vi "Lockin-4461_Multiple Inputs and Outputs_KH_functional_global_waveform.vi"(8 "stop":bool) -> ()   [LabVIEW 2013]
uses:
  <vilib>/Analysis/4window.llb/windowTd.ctl
  <vilib>/Analysis/3filter.llb/Filter Structure Type.ctl
  <vilib>/Analysis/baseanly.llb/Mean (DBL).vi
  <vilib>/Analysis/2dsp.llb/Decimate (single shot, DBL).vi
  <vilib>/DAQmx/write.llb/DAQmx Write (Analog 1D Wfm NChan NSamp).vi
  DAQ-Lockin-SubVI/Lock-in Globles Multiple Inputs and Outputs used with FGV.vi
  <vilib>/DAQmx/miscellaneous.llb/DAQmx Fill In Error Info.vi
  <vilib>/measure/macond.llb/IIR Filter for N Chan.vi
  <vilib>/measure/madcrms.llb/Basic Averaged DC-RMS for N Chan.vi
  <vilib>/measure/maspectr.llb/FFT Power Spectrum and PSD for N Chan.vi
  <vilib>/Analysis/NI_AALPro.lvlib
  <vilib>/Analysis/NI_AALBase.lvlib
  <vilib>/measure/NI_MAPro.lvlib
  <vilib>/measure/NI_MABase.lvlib
panel:
  out "phase log":dbl[](array[numeric])=[0.9999999998974775, 0.9999999998974775, 0.9999999998974775, 0.9999999998974775]
  in  "Input Signals":i16(slide)=2 scale=1.0..20.0
  in  "Tab Control 2":T1(tab)=enum."Lock-in Settings"
  in  "Auto control  max AI rate/ AI block size":bool=TRUE
  in  "AI Buffer Size (S)":i32=10
  in  "AI Block Size":i32=14350
  out "AI Rate":dbl=193151.0 format="%.2f"
  in  "AI Configuration":T2(array[cluster])=[{"AI.Coupling"=10050, "AI.Max"=10.0, "AI.Min"=-10.0, "Input physical channels"="PXI1Slot2/ai0:1"}, {"AI.Coupling"=10050, "AI.Max"=10.0, "AI.Min"=-10.0, "Input physical channels"="PXI1Slot3/ai0:1"}, {"AI.Coupling"=10050, "AI.Max"=10.0, "AI.Min"=-10.0, "Input physical channels"="PXI1Slot5/ai0:1"}, {"AI.Coupling"=10050, "AI.Max"=10.0, "AI.Min"=-10.0, "Input physical channels"="PXI1Slot6/ai0:1"}] {"AI.Coupling" items=["AC"=10045, "DC"=10050, "GND"=10066]}
  in  "AO Configuration":T3(array[cluster])=[{"Output physical channels"="PXI1Slot2/ao0:1", "AO. Max"=0.1, "AO.Min"=-0.1}, {"Output physical channels"="PXI1Slot3/ao0:1", "AO. Max"=0.25, "AO.Min"=-0.25}, {"Output physical channels"="PXI1Slot5/ao0:1", "AO. Max"=0.1, "AO.Min"=-0.1}, {"Output physical channels"="PXI1Slot6/ao0:1", "AO. Max"=0.1, "AO.Min"=-0.1}]
  in  "OSC Configuration":T4(array[cluster])=[[{"Signal Type"=enum."Sine Wave", "DC"=0.0, "Amplitude"=0.0, "frequency"=13.46, "Phase"=0.0}, {"Signal Type"=enum."Sine Wave", "DC"=0.0, "Amplitude"=0.0005, "frequency"=13.46, "Phase"=0.0}], [{"Signal Type"=enum."Sine Wave", "DC"=0.0, "Amplitude"=0.0, "frequency"=13.46, "Phase"=0.0}, {"Signal Type"=enum."Sine Wave", "DC"=0.0, "Amplitude"=0.0, "frequency"=13.46, "Phase"=0.0}], [{"Signal Type"=enum."Sine Wave", "DC"=0.0, "Amplitude"=0.0, "frequency"=13.46, "Phase"=0.0}, {"Signal Type"=enum."Sine Wave", "DC"=0.0, "Amplitude"=0.0, "frequency"=13.46, "Phase"=0.0}], [{"Signal Type"=enum."Sine Wave", "DC"=-0.0467, "Amplitude"=0.0, "frequency"=13.46, "Phase"=0.0}, {"Signal Type"=enum."Sine Wave", "DC"=0.0, "Amplitude"=0.0, "frequency"=13.46, "Phase"=0.0}]] {"frequency" step=0.001 format="%.3p"; "Amplitude" format="%0.2p"; "DC" min=-0.99 max=0.99 format="%.2p"}
  in  "Phase&Tc":T5(array[cluster])=[{"Phase"=0.0, "Time constant"=0.5, "Set Tc"=FALSE, "Autophase"=FALSE, "Order"=0.0}, {"Phase"=0.0, "Time constant"=0.5, "Set Tc"=FALSE, "Autophase"=FALSE, "Order"=0.0}, {"Phase"=0.0, "Time constant"=0.5, "Set Tc"=FALSE, "Autophase"=FALSE, "Order"=0.0}, {"Phase"=0.0, "Time constant"=0.5, "Set Tc"=FALSE, "Autophase"=FALSE, "Order"=0.0}, {"Phase"=0.0, "Time constant"=0.5, "Set Tc"=FALSE, "Autophase"=FALSE, "Order"=0.0}, {"Phase"=0.0, "Time constant"=0.5, "Set Tc"=FALSE, "Autophase"=FALSE, "Order"=0.0}, {"Phase"=0.0, "Time constant"=0.5, "Set Tc"=FALSE, "Autophase"=FALSE, "Order"=0.0}, {"Phase"=0.0, "Time constant"=0.5, "Set Tc"=FALSE, "Autophase"=FALSE, "Order"=0.0}] {"Phase" min=0.0 max=360.0 scale=0.0..360.0}
  in  "Gain":dbl[](array[numeric])=[0.001, 2e-08, 0.001, 0.001, 0.001, 2e-08]
  in  "frequency":dbl
  out "max ai rate":i32=200000
  in  "zero offset":bool
  in  "measure offset":bool
  out "elapsed time":dbl format="%.2g"
  out "Display 2":string="-189.706780      pA"
  out "Display 1":string="-  1.195069      nA"
  in  "Remote":bool=TRUE
  in  "Display":u16(ring) items=["X and Y", "R and Theta"]
  out "Backlog":u8(slide) scale=0.0..100.0
  out "Sampling information":cluster{"Fs":dbl, "#s":dbl}[](array[cluster])=[{"Fs"=193151.0, "#s"=14350.0}, {"Fs"=193151.0, "#s"=14350.0}, {"Fs"=193151.0, "#s"=14350.0}, {"Fs"=193151.0, "#s"=14350.0}]
  out "AO Task":refnum<k21>[](array[refnum])
  out "AI task":refnum<k21>[](array[refnum])
  in  "Tab Control":T6(tab)=enum."Input signals"
  out "Display X (or R) A":dbl[](graph)=[0.0003515597766155211, 0.0003507181675748926, 0.00035141371795365553, 0.0003511676429896116, 0.00035187230028368424, 0.00035142951363845783, 0.00035200218342147584, 0.0003516475669745772, 0.0003513264804061819, 0.0003512466291338144, 0.00035057064868592705, 0.0003509796679868739, 0.0003503537452691344, 0.00035135722504198624, 0.0003499281739531895, 0.00035086727974118317, 0.00035123877543565506, 0.00035105622304100427, 0.00035125795255371527, 0.00035135096570343606, 0.00035150903711195496, 0.0003505963637110228, 0.00035169258826266966, 0.00035039322315619063, 0.00035053162210950205, 0.00034979480515196903, 0.00035116833497217555, 0.00035144449100699994, 0.0003510879884516026, 0.00035159349196440626, 0.0003508268451218459, 0.0003511494372195583, 0.0003501864505254134, 0.00035068434585759, 0.0003499157469483272, 0.00035133561940496534, 0.0003501980965627419, 0.0003508062229105727, 0.0003512488754734741, 0.00035101108207568276, 0.000350758527959875, 0.0003505205072637121, 0.0003508151287793871, 0.0003508447380896511, 0.0003507555783012489, 0.0003502437335620398, 0.00035109131124810123, 0.0003498450741887054, 0.00035085670677781735, 0.00034947118732054223, 0.0003511126940251815, 0.0003498712344731183, 0.00035107848043918404, 0.00035092762190149656, 0.00035131019104293144, 0.00035117278992843757, 0.00035060771724494964, 0.00035097354822363525, 0.00034979186802935094, 0.0003511746212457802, 0.0003504305912612818, 0.0003514156401972867, 0.0003503117115571819, 0.0003512893859642446, 0.0003509935260745274, 0.0003513343838004985, 0.00035176841277986657, 0.0003515970316337863, 0.0003513166742771524, 0.00035104054487817416, 0.0003513553972404074, 0.0003509590909684851, 0.00035237906837522605, 0.00034999762062152867, 0.00035101065218240423, 0.0003504366384126203, 0.00035118217997485036, 0.00035142807787819834, 0.00035048373763264237, 0.00035091253545080304, 0.00035015216674575555, 0.00035129179836784774, 0.00035001054715737636, 0.0003513927563841236, 0.0003506721750452684, 0.00035171243027286867, 0.0003514132808403294, 0.00035144774997313054, 0.00035154044709008854, 0.0003519234717441954, 0.0003516730726749858, 0.0003510679416845872, 0.00035125236026625956, 0.0003506717477152614, 0.00035179090850881385, 0.00035059443995565375, 0.0003512356648576366, 0.00035099014639157884, 0.00035160877389527615, 0.0003511922254044786, 0.0003522473208559999, 0.000351701222721286, 0.00035138480038931065, 0.0003513741316379797, 0.0003514851249003675, 0.00035153133788109374, 0.00035099743725480883, 0.0003517112066303713, 0.00035087507155982204, 0.0003514136294778693, 0.00035113141545342375, 0.0003516959886248813, 0.00035089134479069386, 0.00035195932575444284, 0.0003510852464980746, 0.00035095112846043197, 0.00035142787266349444, 0.00035033572449709563, 0.0003518389763278957, 0.0003509974314077956, 0.0003521376695816606, 0.0003512642342070748, 0.00035127618489995405, 0.0003514483445065015, 0.00035163795610624693, 0.00035111410128884024, 0.0003509321167631999, 0.0003510796360339337, 0.0003503292989579528, 0.00035156402647202597, 0.0003512873517971787, 0.00035157967118798955, 0.0003510116552725674, 0.00035141232666041183, 0.00035107492263834197, 0.0003512565883348785, 0.0003508476519342546, 0.00035108010765180813, 0.0003516328893962722, 0.00035126967501414075, 0.00035163302601165687, 0.0003503689014483799, 0.00035132816396016856, 0.00035068072793987285, 0.00035165998148334955, 0.0003506716705224395, 0.00035129129082704685, 0.0003506971941344991, 0.000350963932032198, 0.00035118513223693614, 0.00035074827788279046, 0.0003510020040280428, 0.0003504848068533489, 0.0003513321853419367, 0.0003503106012231704, 0.00035095822008976673, 0.0003502387857211528, 0.00035109477850426885, 0.0003507864147016284, 0.00035140137858089053, 0.0003514994969105284, 0.0003513918557124627, 0.0003513696821528527, 0.0003508483346289989, 0.0003515212484504822, 0.0003510208186503463, 0.00035172200150656446, 0.00035110641441137973, 0.00035150387093385414, 0.000351046214234429, 0.0003512959219150425, 0.00035191226359241245, 0.0003519236956018965, 0.0003521320087141144, 0.00035099481829272187, 0.00035189540980659097, 0.00035122584644459046, 0.00035158482485956113, 0.0003502803891156385, 0.00035140356164375307, 0.0003509192077086382, 0.0003516851651443288, 0.00035113340325199413, 0.0003512155559510749, 0.0003512258338077835, 0.0003520237023195563, 0.00035088778042110256, 0.00035164083859914543, 0.0003511937863128998, 0.0003518097746241161, 0.0003512714055365024, 0.000352054622085523, 0.0003513780489555605, 0.0003520135769537603, 0.00035157613181737254, 0.0003514540449784146, 0.00035148596975263194, 0.00035058490211263083, 0.0003514386933989605, 0.0003509759320918032]
  out "Display Y (or Theta) A":dbl[](graph)=[-6.733399539668474e-05, -6.542411496845478e-05, -6.796694874685229e-05, -6.507135674382902e-05, -6.76731893269279e-05, -6.432724937539189e-05, -6.686858480018215e-05, -6.439302698787755e-05, -6.743074524483553e-05, -6.5540559290562e-05, -6.769912727311773e-05, -6.675855899422707e-05, -6.556455830757394e-05, -6.791926016049456e-05, -6.499870275650685e-05, -6.76094096444829e-05, -6.409372415827203e-05, -6.690358743848511e-05, -6.376319395976735e-05, -6.661678688045064e-05, -6.475221640770524e-05, -6.767037729114109e-05, -6.65568517718371e-05, -6.61078983653106e-05, -6.72090065494324e-05, -6.491767883192775e-05, -6.840639245595013e-05, -6.446292181235111e-05, -6.733865135996714e-05, -6.40653784901512e-05, -6.70766205814384e-05, -6.448431014524983e-05, -6.721244620921082e-05, -6.59878655486392e-05, -6.692322551150028e-05, -6.69019264583306e-05, -6.53521862403277e-05, -6.794558923933263e-05, -6.499376607325872e-05, -6.696965991750598e-05, -6.461599929467364e-05, -6.687775724991745e-05, -6.35960014145792e-05, -6.71748832581576e-05, -6.492398900048032e-05, -6.746798157246069e-05, -6.634689247733003e-05, -6.592248825579343e-05, -6.76983125588508e-05, -6.466202421410609e-05, -6.750345332833928e-05, -6.450271804110632e-05, -6.73820213196671e-05, -6.398878990855814e-05, -6.699882608984017e-05, -6.499280498169577e-05, -6.738425010553764e-05, -6.660128249440328e-05, -6.641623559943719e-05, -6.741839015150833e-05, -6.490399197802229e-05, -6.807262637843706e-05, -6.461095964170923e-05, -6.741693933791136e-05, -6.396241139824065e-05, -6.68953533836962e-05, -6.437486412654718e-05, -6.719672530343625e-05, -6.601025951582242e-05, -6.755243507643756e-05, -6.683904754234452e-05, -6.581328668735525e-05, -6.7956730495926e-05, -6.454210702322087e-05, -6.700846714162137e-05, -6.487036358948187e-05, -6.717145047610366e-05, -6.394657730710213e-05, -6.721398561579939e-05, -6.542844878392274e-05, -6.72242800275423e-05, -6.601836591155777e-05, -6.679640312152599e-05, -6.724964008795247e-05, -6.524389201445212e-05, -6.81709788892876e-05, -6.504870506524659e-05, -6.716417310946288e-05, -6.469364606167295e-05, -6.64118927639841e-05, -6.428422401809015e-05, -6.726075100677492e-05, -6.602001398773281e-05, -6.684946783051746e-05, -6.665356018961591e-05, -6.559302821306713e-05, -6.823961541895857e-05, -6.489902378019219e-05, -6.747231633806965e-05, -6.460461787722171e-05, -6.739619325891061e-05, -6.42568749063365e-05, -6.728357578332122e-05, -6.572581320455293e-05, -6.733133575279844e-05, -6.745384605205556e-05, -6.654768580556922e-05, -6.752884945881219e-05, -6.516474446690376e-05, -6.800609459823608e-05, -6.47878614014136e-05, -6.730160658797204e-05, -6.420250070636625e-05, -6.676581343835398e-05, -6.447454426249553e-05, -6.739644425949934e-05, -6.633928104016707e-05, -6.668506011610336e-05, -6.704708770176857e-05, -6.518924517552728e-05, -6.80110716513718e-05, -6.449044290923919e-05, -6.713463098761624e-05, -6.431427908560736e-05, -6.666702370071547e-05, -6.380160055564429e-05, -6.69295226583365e-05, -6.559831844106169e-05, -6.733302905782082e-05, -6.676258268638944e-05, -6.581664753168712e-05, -6.791627178025961e-05, -6.483985086130437e-05, -6.771582429628417e-05, -6.456692771022534e-05, -6.710554331363558e-05, -6.416205680544463e-05, -6.721382973122853e-05, -6.497521331755278e-05, -6.762221774081424e-05, -6.644148745970977e-05, -6.650204706057299e-05, -6.779409446006897e-05, -6.513429971844772e-05, -6.716283035881229e-05, -6.500520220536936e-05, -6.748818593189037e-05, -6.375021526081944e-05, -6.679304519274533e-05, -6.44009832356367e-05, -6.697029619860621e-05, -6.614507717764695e-05, -6.675045380090485e-05, -6.699368958403159e-05, -6.540977419016514e-05, -6.751824094235534e-05, -6.497224203386006e-05, -6.747996187391402e-05, -6.445371747351958e-05, -6.694216412544935e-05, -6.39145549472495e-05, -6.67208337122775e-05, -6.499887641961741e-05, -6.75636406906266e-05, -6.646187561893783e-05, -6.6422353672184e-05, -6.774188283466967e-05, -6.49718493653088e-05, -6.774060340062207e-05, -6.447729538855726e-05, -6.7276329542447e-05, -6.45413468122233e-05, -6.725796598454556e-05, -6.43215545435326e-05, -6.710426281533913e-05, -6.640793922515245e-05, -6.688725807556598e-05, -6.702595030422637e-05, -6.555532275656158e-05, -6.775334049196785e-05, -6.485489689304207e-05, -6.778283710493148e-05, -6.47406497658257e-05, -6.667061103568536e-05, -6.71178176816977e-05, -6.545036016336727e-05, -6.758648874374465e-05, -6.648186107488955e-05, -6.564351224820166e-05, -6.726344507999936e-05, -6.562770441403993e-05, -6.793015780847218e-05, -6.469220243177453e-05, -6.740767551952607e-05, -6.44720529171589e-05, -6.682838905210087e-05, -6.483406975990464e-05, -6.710332224721377e-05, -6.629467593853179e-05, -6.657765389063085e-05]
  in  "long term averaging type":enum16{"Linear", "Exponential"}(ring)
  in  "averaging type":enum16{"Linear", "Exponential"}(ring)
  out "Waveform Graph":waveform(dbl)[](graph)
  in  "Stream to disk?":bool
  in  "decimating factor":i32
  in  "decimating factor 2":i32=1
  out "Waveform Graph 2":cluster{"f0":dbl, "df":dbl, "magnitude":dbl[]}[](graph)
  in  "window":T7=1 items=["Rectangle"=0, "Hanning"=1, "Hamming"=2, "Blackman-Harris"=3, "Exact Blackman"=4, "Blackman"=5, "Flat Top"=6, "4 Term B-Harris "=7, "7 Term B-Harris"=8, "Low Sidelobe"=9, "Blackman Nuttall"=11, "Triangle"=30, "Bartlett-Hanning"=31, "Bohman"=32, "Parzen"=33, "Welch"=34, "Kaiser"=60, "Dolph-Chebyshev"=61, "Gaussian"=62]
  in  "averaging parameters":T8={"averaging mode"=enum."No averaging", "weighting mode"=enum."Exponential", "number of averages"=10} {"number of averages" min=1}
  in  "dB On (F)":bool
  out "Results (X, Y, R, Theta)":dbl[][](array[numeric]) format="%#_6p"
  out "Measure?":u16[](array[numeric])=[2, 1, 2, 2, 2, 1]
  in  "Cluster (unused right now)":T9={"Amplitude"=[0.001, 2e-08, 0.001, 0.001, 0.001, 2e-08], "DC"=[0.001, 2e-08, 0.001, 0.001, 0.001, 2e-08], "phase"=[0.001, 2e-08, 0.001, 0.001, 0.001, 2e-08], "Array"=[]}
  out "offsets":dbl[](array[numeric])
  in  "IIR filter specifications":T10={"Topology"=enum."Butterworth", "Type"=enum."Lowpass", "Order"=1, "Lower Fc"=100.0, "Upper Fc"=200.0, "PB Ripple"=1.0, "SB Attenuation"=60.0} {"PB Ripple" format="%0.2f"; "SB Attenuation" format="%0.2f"; "Lower Fc" format="%0.2p"; "Upper Fc" format="%0.2p"}
  in  "filter structure option":T11=10 items=["IIR 2nd Order"=0, "IIR 4th Order"=1, "Auto Select"=10]
  in  "reset filters":bool
  out "Waveform Chart":dbl[][](graph)
  # "*****Customized for 4461 + 4462 cards; functional globals*****"
  # "Real time Adjustable Values"
  # "Configurations"
  # "should this be x multiple\nof the frequency?"
  # "The top array index selects which card you are setting the outputs for,and the second index selects which output chanel on that card.\n\nFor Phase&Tc, you must have an array element initialized for each input signal."
  # "Features:\n1, Any number of input and output channels\n2, Each AO outputs an DC+AC signal, DC for sample biasing and AC for OSC. These values can be adjusted in real time.\n3, Synchronous filtering\n\nInstructions:\n1, Array index of AI configuration and AO configuration refers to task.\n2, Array index in Amplifier Settings, Phase$&Tc control , and gains correlates to channel number.\n3, Each 4461 board can have 2 lock-in channels. Syntax for 2 channles, e.g. PXI1Slot2/ai0:1. If you want to use just one, then PXI1Slot2/ai0.\n4, Parameters (especially DC value for sample biasing) can be remotely controlled by clicking \"local\"and \"remote\" button. In real experiments, put golable values (can be found in Lock-in globles.vi) in your VI to control the lock-in and read out.\n5, choose OSC frequencies to be multiple of \nAI Rate/AI Block SIze to have best performance.\n\n-Guanglei 06/23/2011\n\nUpdate:\n1. Allows any number of lockin amplifiers and AO tasks.\n2. Delete the channels from any AI/AO Configuration elements you do not want to use.\n3. Rows (first index) of the OSC Configuration correspond to different AO tasks, while columns (second index) correspond to AO channels in that task. All channels in a given element of the AO Configuration array will go into a single task.\n4. The same number of output channels must go in each AO task.\n5. Make sure a Phase&Tc element and an Amplifier Settings element is set for each AI channel.\n-Joe 12/3/2013"
  # "hide stuff here in this tab"
  # "multiple of frequency??"
  # "this is \"time constant\""
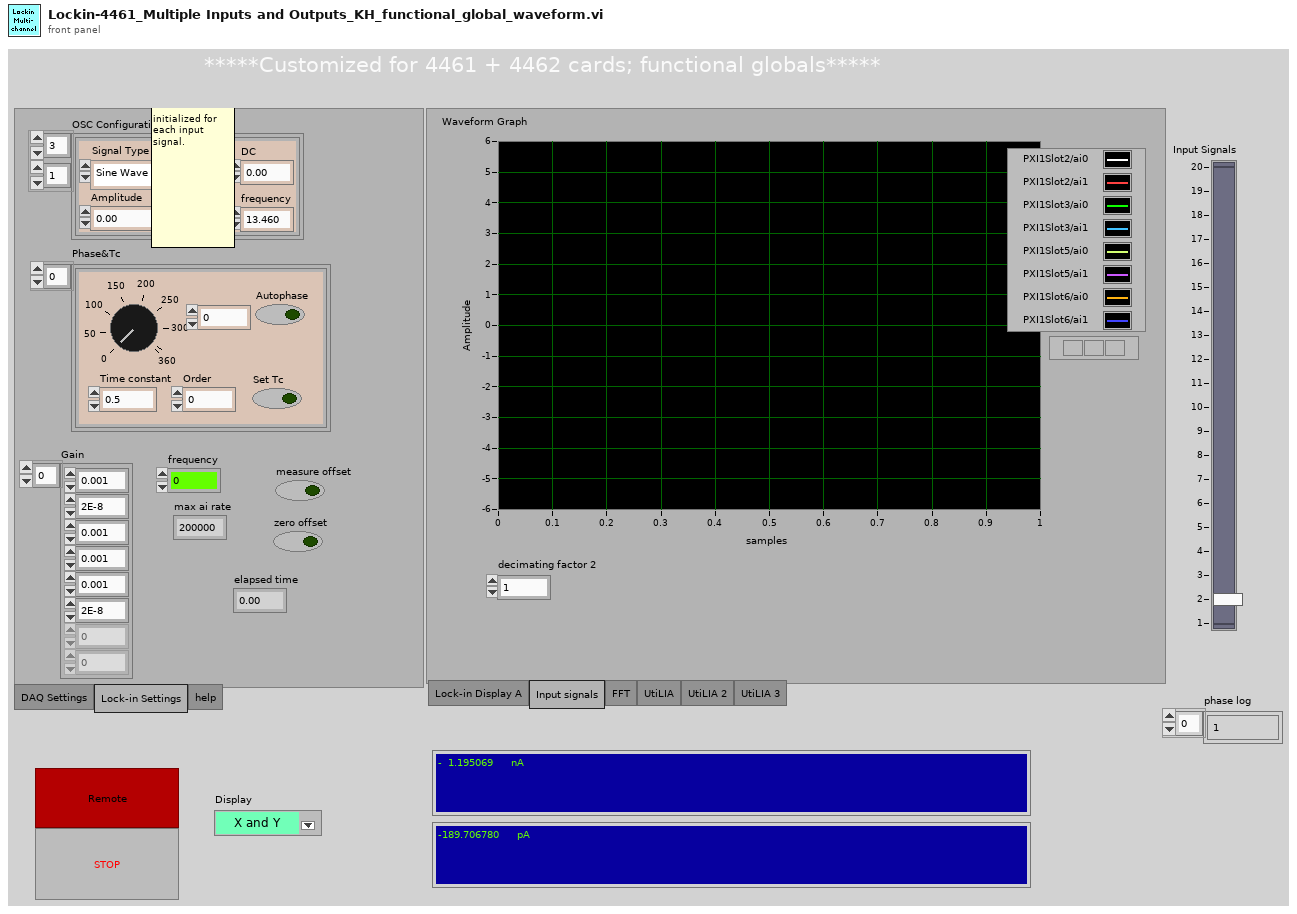
[diagram p1: front panel]
types:
  T1 = enum32{"DAQ Settings", "Lock-in Settings", "help"}
  T2 = cluster{"AI.Coupling":i32, "AI.Max":dbl, "AI.Min":dbl, "Input physical channels":tag}[]
  T3 = cluster{"Output physical channels":tag, "AO. Max":dbl, "AO.Min":dbl}[]
  T4 = cluster{"Signal Type":enum16{"Sine Wave", "Triangle Wave", "Square Wave", "Sawtooth Wave"}, "DC":dbl, "Amplitude":dbl, "frequency":dbl, "Phase":dbl}[][]
  T5 = cluster{"Phase":dbl, "Time constant":dbl, "Set Tc":bool, "Autophase":bool, "Order":dbl}[]
  T6 = enum32{"Lock-in Display A", "Input signals", "FFT", "UtiLIA", "UtiLIA 2", "UtiLIA 3"}
  T7 = typedef "NI_AALPro.lvlib/windowTd.ctl" = u32
  T8 = cluster{"averaging mode":enum16{"No averaging", "Vector averaging", "RMS averaging", "Peak hold"}, "weighting mode":enum16{"Linear", "Exponential"}, "number of averages":u32}
  T9 = cluster{"Amplitude":dbl[], "DC":dbl[], "phase":dbl[], "Array":enum16{"Sine Wave", "Triangle Wave", "Square Wave", "Sawtooth Wave"}[]}
  T10 = cluster{"Topology":enum16{"Off", "Butterworth", "Chebyshev", "Inverse Chebyshev", "Elliptic", "Bessel"}, "Type":enum16{"Lowpass", "Highpass", "Bandpass", "Bandstop"}, "Order":i32, "Lower Fc":dbl, "Upper Fc":dbl, "PB Ripple":dbl, "SB Attenuation":dbl}
  T11 = typedef "NI_AALBase.lvlib/Filter Structure Type.ctl" = u16
  T12 = cluster{"Signal Type":enum16{"Sine Wave", "Triangle Wave", "Square Wave", "Sawtooth Wave"}, "DC":dbl, "Amplitude":dbl, "frequency":dbl, "Phase":dbl}
  T13 = enum16{"Sine Wave", "Triangle Wave", "Square Wave", "Sawtooth Wave"}
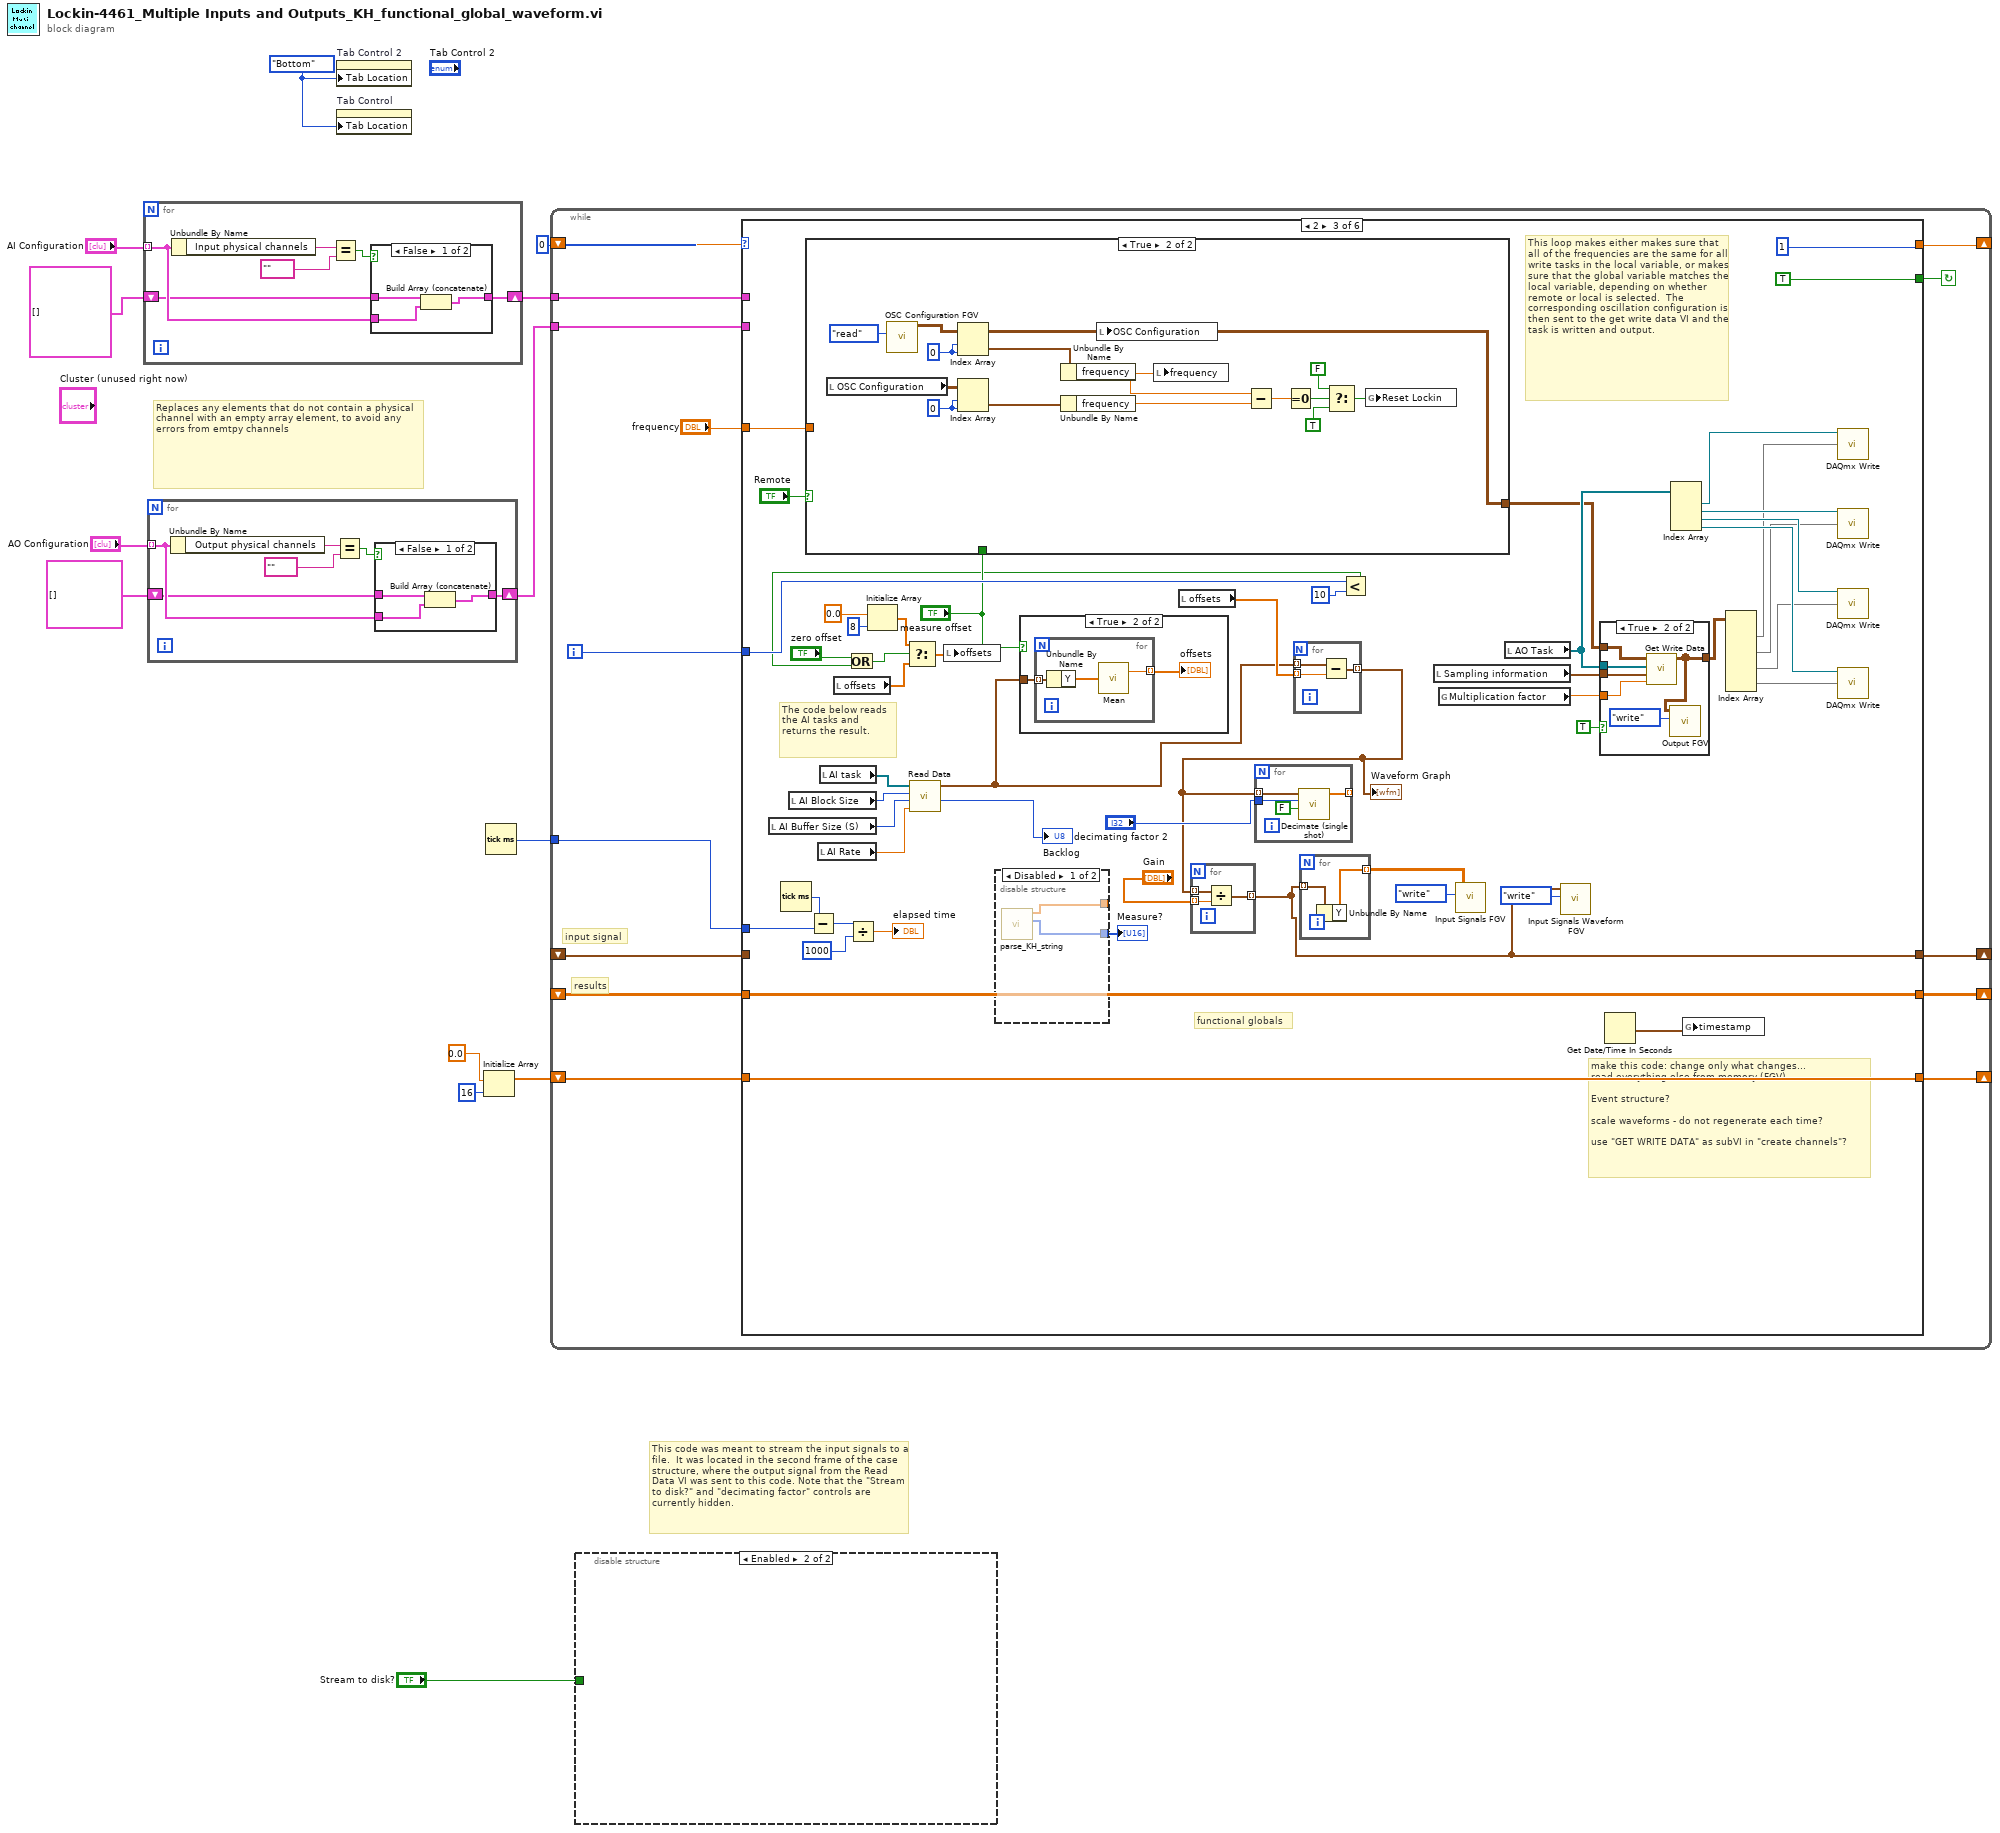
[diagram p0: block diagram]
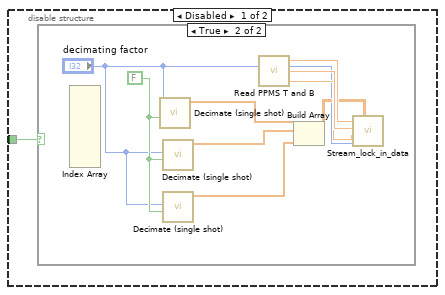
[diagram p2: hidden frame]
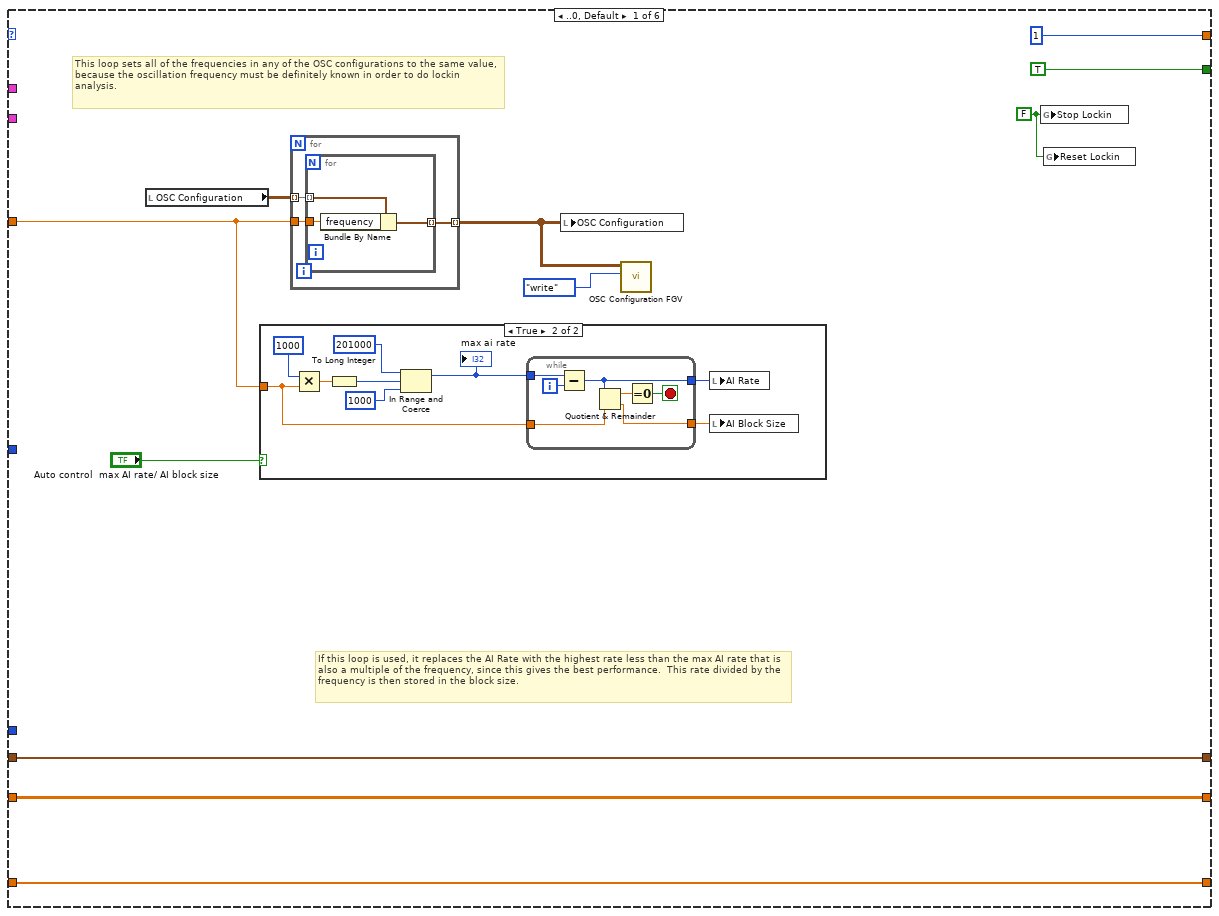
[diagram p6: hidden frame]
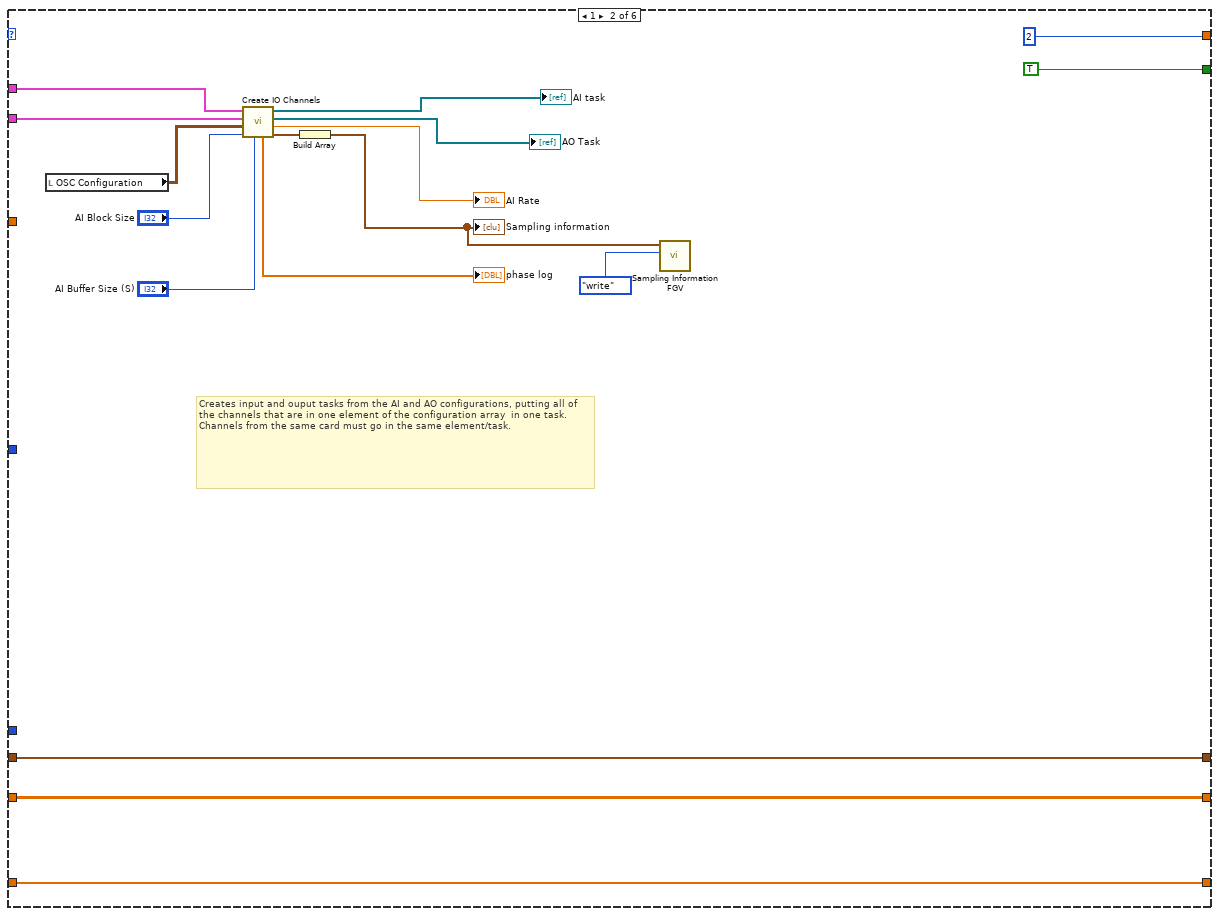
[diagram p8: hidden frame]
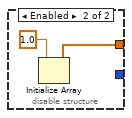
[diagram p10: hidden frame]
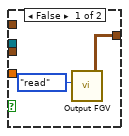
[diagram p11: hidden frame]
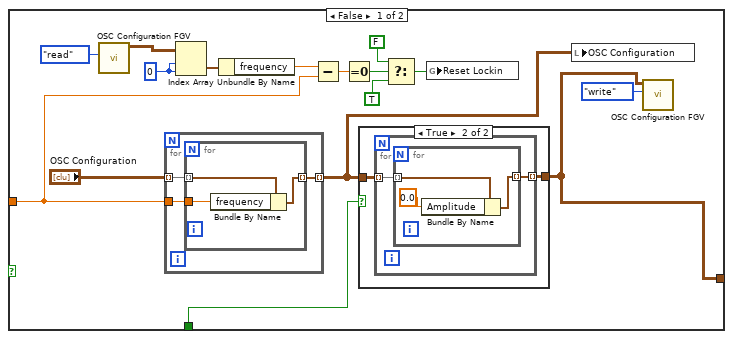
[diagram p12: hidden frame]
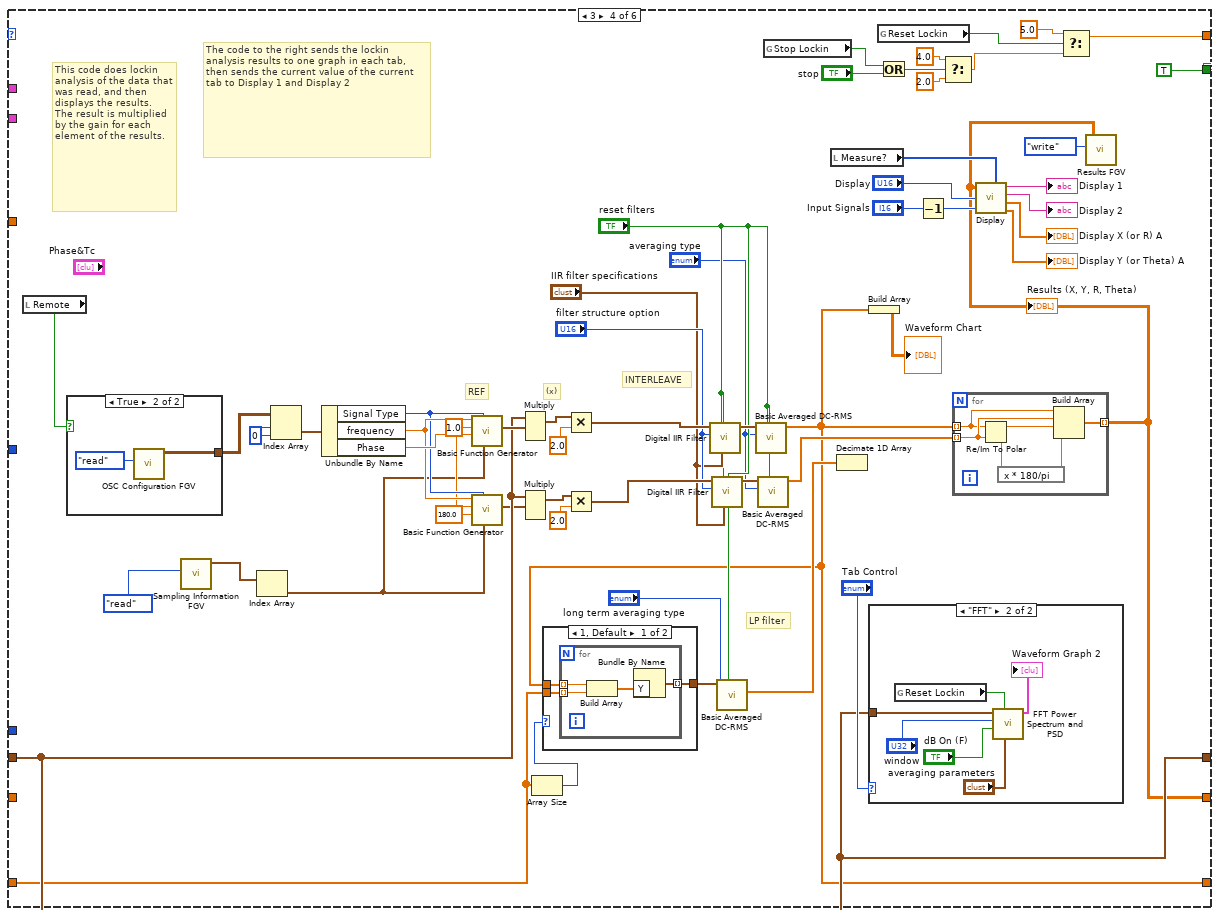
[diagram p14: hidden frame]
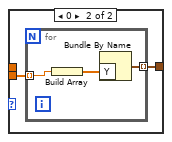
[diagram p15: hidden frame]
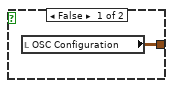
[diagram p17: hidden frame]
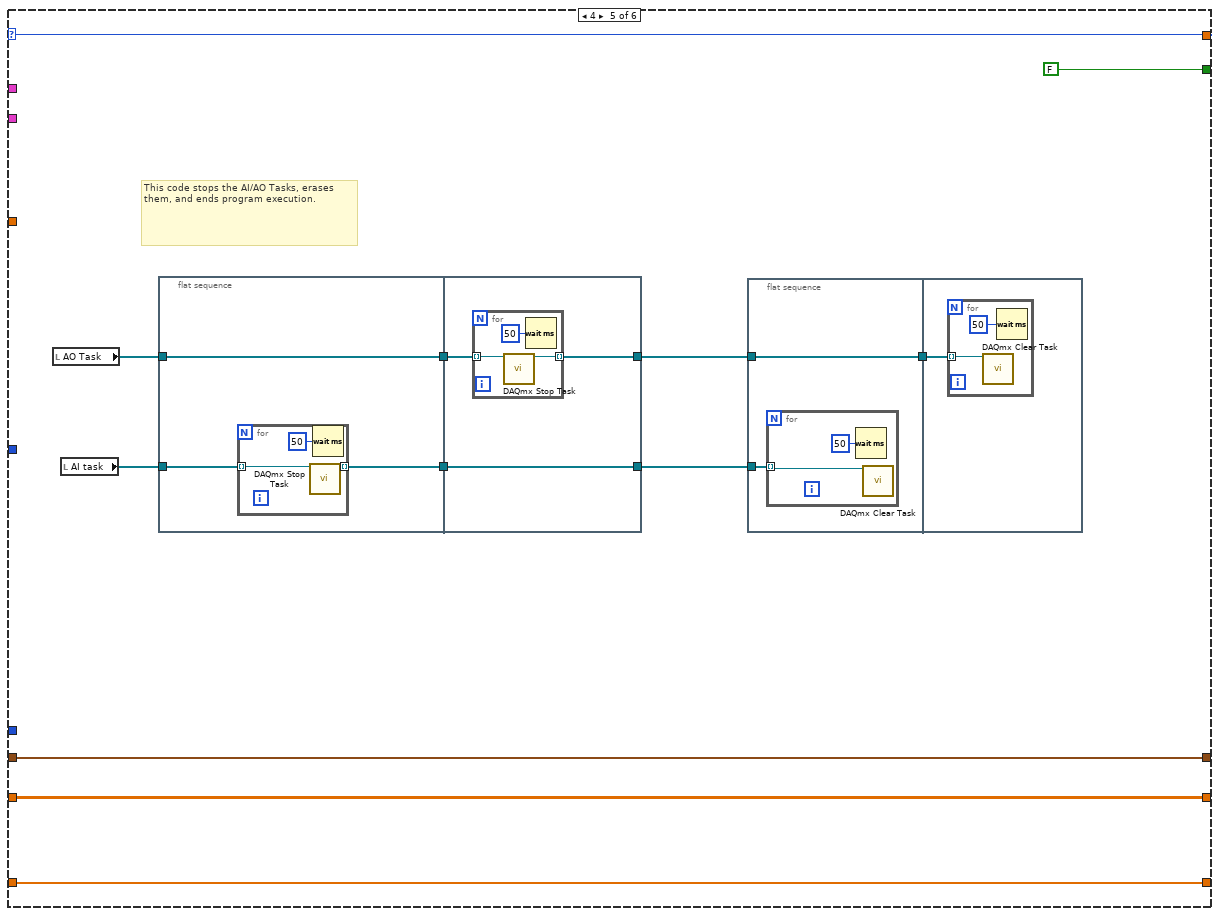
[diagram p18: hidden frame]
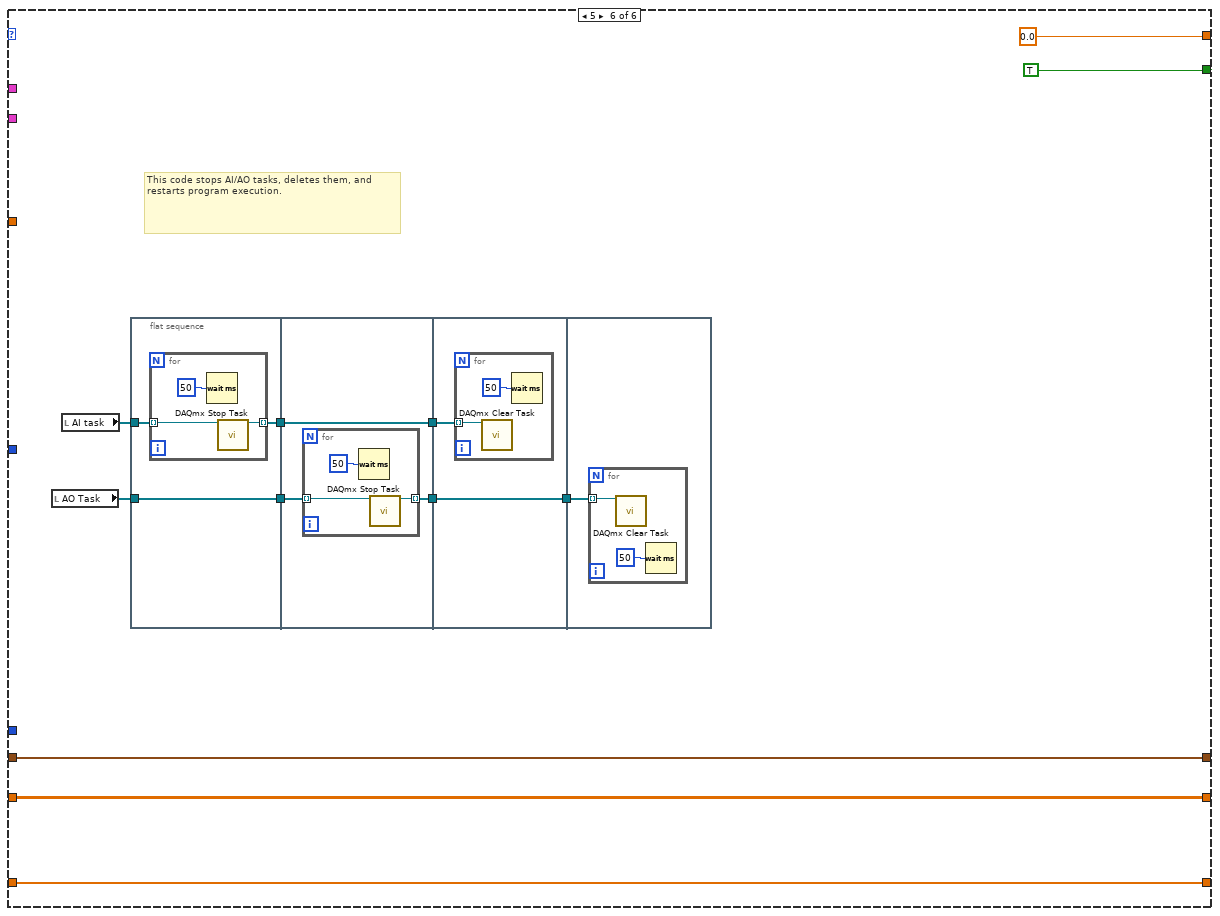
[diagram p19: hidden frame]
diagram:
  w7 = enum32{"Top", "Bottom", "Left", "Right"}."Bottom" ("Tab Location")
  # "This code was meant to stream the input signals to a file.  It was located in the second frame of the case structure, where the output signal from the Read Data VI was sent to this code. Note that the \"Stream to disk?\" and \"decimating factor\" controls are currently hidden."
  # "Replaces any elements that do not contain a physical channel with an empty array element, to avoid any errors from emtpy channels"
  n1 = for {
    tunnel: "AI Configuration" -> [w16] mode=indexing
    shift-right: [w14] -> w13
    shift-left: T2 [] ("AI Configuration") -> [w15]
    n2 = Unbundle By Name(w16) -> ("Input physical channels"=w18:tag)
    n3 = Equal?(x=w18, y=tag "" ("Empty physical channels")) -> (x = y?=w19:bool)
    n4 = case shown="False" w19 {
      tunnel: w16 -> [w21 _]
      tunnel: w15 -> [w22 w23]
      tunnel: [w20 w23] -> w14
      frame False {
        n5 = Build Array (concatenate)(w22, w21) -> (w20:T2)
      }
      frame True {
      }
    }
  }
  n6 = for {
    tunnel: "AO Configuration" -> [w26] mode=indexing
    shift-right: [w24] -> w5
    shift-left: T3 [] ("AO Configuration 2") -> [w25]
    n7 = Unbundle By Name(w26) -> ("Output physical channels"=w28:tag)
    n8 = Equal?(x=w28, y=tag "" ("Empty physical channels")) -> (x = y?=w29:bool)
    n9 = case shown="False" w29 {
      tunnel: w26 -> [w31 _]
      tunnel: w25 -> [w32 w33]
      tunnel: [w30 w33] -> w24
      frame False {
        n10 = Build Array (concatenate)(w32, w31) -> (w30:T3)
      }
      frame True {
      }
    }
  }
  n11 = property on="Tab Control 2" class="TabCtl (strict)"("Tab Location"=w7) -> ()  [unwired: 2 in, 2 out]
  n12 = property on="Tab Control" class="TabCtl (strict)"("Tab Location"=w7) -> ()  [unwired: 2 in, 2 out]
  n13 = Initialize Array(0.0, 16 ("dimension size")) -> (w3:dbl[])
  n14 = Tick Count (ms)() -> (millisecond timer value=w1:u32)
  n15 = while {
    shift-right: [w47] -> _
    shift-left: 0 -> [w46]
    tunnel: w13 -> [w45]
    tunnel: w5 -> [w43]
    shift-right: [w42] -> _
    shift-left: _ -> [w41]
    shift-right: [w39] -> _
    shift-left: _ -> [w40]
    shift-right: [w37] -> _
    shift-left: w3 -> [w36]
    tunnel: w1 -> [w34]
    i -> [w38]
    stop <- w44 continue-if-true
    # "results"
    # "input signal"
    n16 = case shown="2" w46 {
      selector: w46 -> [_ _ _ _ w315 _]
      tunnel: [1 2 1 w269 w315 0.0 ("f")] -> w47
      tunnel: w45 -> [_ w92 _ _ _ _]
      tunnel: [TRUE TRUE TRUE TRUE FALSE TRUE] -> w44
      tunnel: w43 -> [_ w91 _ _ _ _]
      tunnel: [w51 w86 w105 w247 w307 w338] -> w42
      tunnel: w41 -> [w51 w86 _ w247 w307 w338]
      tunnel: w40 -> [w50 w85 w127 _ w306 w337]
      tunnel: [w50 w85 w127 w244 w306 w337] -> w39
      tunnel: w38 -> [_ _ w118 _ _ _]
      tunnel: [w49 w82 w123 w223 w305 w336] -> w37
      tunnel: w36 -> [w49 w82 w123 w238 w305 w336]
      tunnel: "frequency" -> [w48 _ w122 _ _ _]
      tunnel: w34 -> [_ _ w101 _ _ _]
      frame ..0, Default {
        w57 = FALSE ("Stop Lockin")
        # "If this loop is used, it replaces the AI Rate with the highest rate less than the max AI rate that is also a multiple of the frequency, since this gives the best performance.  This rate divided by the frequency is then stored in the block size."
        # "This loop sets all of the frequencies in any of the OSC configurations to the same value, because the oscillation frequency must be definitely known in order to do lockin analysis."
        n17 = local read "OSC Configuration"() -> (w54:T4)
        n18 = case shown="True" "Auto control  max AI rate/ AI block size" {
          tunnel: w48 -> [_ w65]
          frame False {
          }
          frame True {
            n19 = Multiply(x=1000, y=w65) -> (x*y=w71:dbl)
            n20 = To Long Integer(number=w71) -> (32bit integer=w69:i32)
            n21 = In Range and Coerce(upper limit=201000, x=w69, lower limit=1000) -> (coerced(x)=w66:i32)  [unwired: 1 out]
            "max ai rate" <- w66
            n22 = while {
              tunnel: w66 -> [w80]
              tunnel: [w78] -> w73
              tunnel: [w76] -> w72
              tunnel: w65 -> [w77]
              i -> [w79]
              stop <- w74 stop-if-true
              n23 = Subtract(x=w80, y=w79) -> (x-y=w76:i32)
              n24 = Quotient & Remainder(x=w76, y=w77) -> (x-y*floor(x/y)=w75:dbl, floor(x/y)=w78:dbl)
              n25 = Equal To 0?(x=w75) -> (x = 0?=w74:bool)
            }
            n26 = local write "AI Rate"(w72) -> ()
            n27 = local write "AI Block Size"(w73) -> ()
          }
        }
        n28 = for {
          tunnel: w54 -> [w61] mode=indexing
          tunnel: [w60] -> w53 mode=indexing
          tunnel: w48 -> [w59]
          n29 = for {
            tunnel: w61 -> [w64] mode=indexing
            tunnel: [w63] -> w60 mode=indexing
            tunnel: w59 -> [w62]
            n30 = Bundle By Name(cluster=w64, "frequency"=w62) -> (w63:T12)
          }
        }
        n31 = local write "OSC Configuration"(w53) -> ()
        n32 = call "OSC Configuration FGV.vi"("Function"=enum16{"write", "read"}."write", "OSC Configuration"=w53) -> ()  [unwired: 4 in, 2 out]
        n33 = global write "Lock-in Globles Multiple Inputs and Outputs used with FGV.vi" "Stop Lockin"(w57) -> ()
        n34 = global write "Lock-in Globles Multiple Inputs and Outputs used with FGV.vi" "Reset Lockin"(w57) -> ()
      }
      frame 1 {
        # "Creates input and ouput tasks from the AI and AO configurations, putting all of the channels that are in one element of the configuration array  in one task.  Channels from the same card must go in the same element/task."
        n35 = local read "OSC Configuration"() -> (w95:T4)
        n36 = call "Create IO Channels.vi"("AI Buffer Size (s)"="AI Buffer Size (S)", "AI Block Size"="AI Block Size", "OSC Configuration"=w95, "AO Configuration"=w91, "AI Configuration"=w92) -> ("sampling info"=w87:cluster{"Fs":dbl, "#s":dbl}, "AI Rate"=→"AI Rate":dbl, "AO Task"=→"AO Task":refnum<k21>[], "AI task"=→"AI task":refnum<k21>[], "phase log"=→"phase log":dbl[])  [unwired: 1 in, 1 out]
        n37 = Build Array(w87) -> (w81:cluster{"Fs":dbl, "#s":dbl}[])
        "Sampling information" <- w81
        n38 = call "Sampling Information FGV.vi"("Function"=enum16{"write", "read"}."write", "Sampling information"=w81) -> ()  [unwired: 4 in, 2 out]
      }
      frame 2 {
        # "make this code: change only what changes...\nread everything else from memory (FGV)\n\nEvent structure?\n\nscale waveforms - do not regenerate each time?\n\nuse \"GET WRITE DATA\" as subVI in \"create channels\"?"
        # "functional globals"
        # "The code below reads the AI tasks and returns the result."
        # "This loop makes either makes sure that all of the frequencies are the same for all write tasks in the local variable, or makes sure that the global variable matches the local variable, depending on whether remote or local is selected.  The corresponding oscillation configuration is then sent to the get write data VI and the task is written and output."
        n39 = local read "AI Buffer Size (S)"() -> (w141:i32)
        n40 = Tick Count (ms)() -> (millisecond timer value=w102:u32)
        n41 = local read "AI Block Size"() -> (w142:i32)
        n42 = case shown="True" "Remote" {
          tunnel: [w179 w209] -> w126
          tunnel: w122 -> [w182 _]
          tunnel: "measure offset" -> [w181 _]
          frame False {
            w191 = 0 ("index")
            n43 = call "OSC Configuration FGV.vi"("Function"=enum16{"write", "read"}."read") -> ("OSC Configuration"=w185:T4)  [unwired: 5 in, 1 out]
            n44 = for {
              tunnel: w182 -> [w205]
              tunnel: "OSC Configuration" -> [w204] mode=indexing
              tunnel: [w203] -> w180 mode=indexing
              n45 = for {
                tunnel: w204 -> [w208] mode=indexing
                tunnel: w205 -> [w207]
                tunnel: [w206] -> w203 mode=indexing
                n46 = Bundle By Name(cluster=w208, "frequency"=w207) -> (w206:T12)
              }
            }
            n47 = Index Array(array=w185, index (row)=w191, index (col)=w191) -> (element=w190:T12)
            n48 = Unbundle By Name(w190) -> ("frequency"=w184:dbl)
            n49 = Subtract(x=w184, y=w182) -> (x-y=w183:dbl)
            n50 = Equal To 0?(x=w183) -> (x = 0?=w189:bool)
            n51 = case shown="True" w181 {
              tunnel: w180 -> [w195 w197]
              tunnel: [w195 w196] -> w179
              frame False {
              }
              frame True {
                n52 = for {
                  tunnel: w197 -> [w199] mode=indexing
                  tunnel: [w198] -> w196 mode=indexing
                  n53 = for {
                    tunnel: w199 -> [w202] mode=indexing
                    tunnel: [w201] -> w198 mode=indexing
                    n54 = Bundle By Name(cluster=w202, "Amplitude"=0.0) -> (w201:T12)
                  }
                }
              }
            }
            n55 = Select(t=FALSE ("Reset Lockin"), s=w189, f=TRUE ("Reset Lockin")) -> (s? t:f=w186:bool)
            n56 = global write "Lock-in Globles Multiple Inputs and Outputs used with FGV.vi" "Reset Lockin"(w186) -> ()
            n57 = local write "OSC Configuration"(w180) -> ()
            n58 = call "OSC Configuration FGV.vi"("Function"=enum16{"write", "read"}."write", "OSC Configuration"=w179) -> ()  [unwired: 4 in, 2 out]
          }
          frame True {
            w219 = 0 ("index")
            w221 = 0 ("index")
            n59 = local read "OSC Configuration"() -> (w211:T4)
            n60 = call "OSC Configuration FGV.vi"("Function"=enum16{"write", "read"}."read") -> ("OSC Configuration"=w209:T4)  [unwired: 5 in, 1 out]
            n61 = Index Array(array=w209, index (row)=w221, index (col)=w221) -> (element=w222:T12)
            n62 = Index Array(array=w211, index (row)=w219, index (col)=w219) -> (element=w218:T12)
            n63 = Unbundle By Name(w222) -> ("frequency"=w210:dbl)
            n64 = Unbundle By Name(w218) -> ("frequency"=w216:dbl)
            n65 = local write "OSC Configuration"(w209) -> ()
            n66 = local write "frequency"(w210) -> ()
            n67 = Subtract(x=w210, y=w216) -> (x-y=w217:dbl)
            n68 = Equal To 0?(x=w217) -> (x = 0?=w215:bool)
            n69 = Select(t=FALSE ("Reset Lockin"), s=w215, f=TRUE ("Reset Lockin")) -> (s? t:f=w212:bool)
            n70 = global write "Lock-in Globles Multiple Inputs and Outputs used with FGV.vi" "Reset Lockin"(w212) -> ()
          }
        }
        n71 = Subtract(x=w102, y=w101) -> (x-y=w100:u32)
        n72 = local read "AI Rate"() -> (w140:dbl)
        n73 = local read "AI task"() -> (w143:refnum<k21>[])
        n74 = local read "offsets"() -> (w116:dbl[])
        n75 = Divide(x=w100, y=u32 1000) -> (x/y=→"elapsed time":dbl)
        n76 = Initialize Array(0.0, 8 ("dimension size")) -> (w113:dbl[])
        n77 = call "Read Data.vi"("AI Rate"=w140, "AI Buffer Size (s)"=w141, "AI Block Size"=w142, "AI task"=w143) -> ("Backlog"=→"Backlog":u8, "Input Signals"=w107:waveform(dbl)[])  [unwired: 5 in, 1 out]
        n78 = disable-structure shown="Disabled" {
          disable-tunnel: [w164 w165] -> _
          disable-tunnel: [w163 _] -> w121
          frame Disabled {
            n79 = call "parse_KH_string.vi"() -> ("Measurement type"=w163:i32[], "Gain"=w164:dbl[])  [unwired: 10 in]
          }
          frame Enabled {
            n80 = Initialize Array(1.0) -> (w165:dbl[])  [unwired: 1 in]
          }
        }
        "Measure?" <- w121
        n81 = case shown="True" "measure offset" {
          tunnel: w107 -> [_ w152]
          frame False {
          }
          frame True {
            n82 = for {
              tunnel: [w156] -> w153 mode=indexing
              tunnel: w152 -> [w155] mode=indexing
              n83 = Unbundle By Name(w155) -> ("Y"=w154:dbl[])
              n84 = call-poly <vilib>:"Mean.vi"("X"=w154) -> ("mean"=w156:dbl)  [unwired: 1 out]
            }
            "offsets" <- w153
          }
        }
        n85 = local read "offsets"() -> (w108:dbl[])
        n86 = for {
          tunnel: w107 -> [w159] mode=indexing
          tunnel: [w158] -> w103 mode=indexing
          tunnel: w108 -> [w157] mode=indexing
          n87 = Subtract(x=w159, y=w157) -> (x-y=w158:waveform(dbl))
        }
        "Waveform Graph" <- w103
        n88 = for {
          tunnel: w103 -> [w162] mode=indexing
          tunnel: [w161] -> w105 mode=indexing
          tunnel: "Gain" -> [w160] mode=indexing
          n89 = Divide(x=w162, y=w160) -> (x/y=w161:waveform(dbl))
        }
        n90 = for {
          tunnel: "decimating factor 2" -> [w170]
          tunnel: w103 -> [w169] mode=indexing
          tunnel: [w168] -> _ mode=indexing
          n91 = call-poly <vilib>:"Decimate (single shot).vi"("averaging"=FALSE, "decimating factor"=w170, "X"=w169) -> ("Decimated Array"=w168:dbl[])  [unwired: 7 in, 1 out]
        }
        n92 = for {
          tunnel: w105 -> [w151] mode=indexing
          tunnel: [w150] -> w106 mode=indexing
          n93 = Unbundle By Name(w151) -> ("Y"=w150:dbl[])
        }
        n94 = Less?(x=w118, y=10) -> (x < y?=w110:bool)
        n95 = Or(x="zero offset", y=w110) -> (x .or. y?=w109:bool)
        n96 = Select(t=w113, s=w109, f=w116) -> (s? t:f=w115:dbl[])
        n97 = local write "offsets"(w115) -> ()
        n98 = local read "Sampling information"() -> (w145:cluster{"Fs":dbl, "#s":dbl}[])
        n99 = global read "Lock-in Globles Multiple Inputs and Outputs used with FGV.vi" "Multiplication factor"() -> (w144:dbl)
        n100 = call "Input Signals FGV.vi"("Function"=enum16{"write", "read"}."write", "Input Signals"=w106) -> ()  [unwired: 4 in, 2 out]
        n101 = local read "AO Task"() -> (w138:refnum<k21>[])
        n102 = call "Input Signals Waveform FGV.vi"("Function"=enum16{"write", "read"}."write", "input signal"=w105) -> ()  [unwired: 4 in, 2 out]
        n103 = case shown="True" TRUE {
          tunnel: w145 -> [_ w178]
          tunnel: w144 -> [_ w176]
          tunnel: w138 -> [_ w177]
          tunnel: [w171 w174] -> w128
          tunnel: w126 -> [_ w175]
          frame False {
            n104 = call "Output FGV.vi"("Function"=enum16{"write", "read"}."read") -> ("Output"=w171:waveform(dbl)[][])  [unwired: 5 in, 1 out]
          }
          frame True {
            n105 = call "Get Write Data.vi"("Multiplication Factor"=w176, "Sampling information 2"=w178, "AO Task"=w177, "OSC Configuration"=w175) -> ("Data"=w174:waveform(dbl)[][])  [unwired: 7 in]
            n106 = call "Output FGV.vi"("Function"=enum16{"write", "read"}."write", "Output"=w174) -> ()  [unwired: 4 in, 2 out]
          }
        }
        n107 = Get Date/Time In Seconds() -> (seconds since 1Jan1904=w146:timestamp)
        n108 = Index Array(array=w138) -> (element #1=w137:refnum<k21>, element #2=w136:refnum<k21>, element #3=w135:refnum<k21>, element #4=w134:refnum<k21>)  [unwired: 4 in]
        n109 = global write "Lock-in Globles Multiple Inputs and Outputs used with FGV.vi" "timestamp"(w146) -> ()
        n110 = Index Array(array=w128) -> (element #1=w133:waveform(dbl)[], element #2=w132:waveform(dbl)[], element #3=w131:waveform(dbl)[], element #4=w130:waveform(dbl)[])  [unwired: 8 in]
        n111 = call-poly <vilib>:"DAQmx Write.vi"("task/channels in"=w137, "data"=w133) -> ()  [unwired: 11 in, 3 out]
        n112 = call-poly <vilib>:"DAQmx Write.vi"("task/channels in"=w136, "data"=w132) -> ()  [unwired: 11 in, 3 out]
        n113 = call-poly <vilib>:"DAQmx Write.vi"("task/channels in"=w135, "data"=w131) -> ()  [unwired: 11 in, 3 out]
        n114 = call-poly <vilib>:"DAQmx Write.vi"("task/channels in"=w134, "data"=w130) -> ()  [unwired: 11 in, 3 out]
      }
      frame 3 {
        w249 = 1.0 ("amplitude")
        w255 = 0 ("disabled index (col)")
        # "INTERLEAVE"
        # "LP filter"
        # "(x)"
        # "REF"
        # "The code to the right sends the lockin analysis results to one graph in each tab, then sends the current value of the current tab to Display 1 and Display 2"
        # "This code does lockin analysis of the data that was read, and then displays the results.  The result is multiplied by the gain for each element of the results."
        n115 = local read "Remote"() -> (w268:bool)
        n116 = case shown="True" w268 {
          tunnel: [w302 w303] -> w256
          frame False {
            n117 = local read "OSC Configuration"() -> (w302:T4)
          }
          frame True {
            n118 = call "OSC Configuration FGV.vi"("Function"=enum16{"write", "read"}."read") -> ("OSC Configuration"=w303:T4)  [unwired: 5 in, 1 out]
          }
        }
        n119 = call "Sampling Information FGV.vi"("Function"=enum16{"write", "read"}."read") -> ("Sampling information"=w242:cluster{"Fs":dbl, "#s":dbl}[])  [unwired: 5 in, 1 out]
        n120 = Index Array(array=w242) -> (element=w241:cluster{"Fs":dbl, "#s":dbl})  [unwired: 1 in]
        n121 = Index Array(array=w256, index (row)=w255, index (col)=w255) -> (element=w254:T12)
        n122 = Unbundle By Name(w254) -> ("Signal Type"=w250:T13, "frequency"=w251:dbl, "Phase"=w253:dbl)
        n123 = call <vilib>:"Basic Function Generator.vi"("sampling info"=w241, "signal type"=w250, "phase"=w253, "amplitude"=w249, "frequency"=w251) -> ("signal out"=w252:waveform(dbl))  [unwired: 4 in, 2 out]
        n124 = call <vilib>:"Basic Function Generator.vi"("sampling info"=w241, "signal type"=w250, "phase"=180.0, "amplitude"=w249, "frequency"=w251) -> ("signal out"=w246:waveform(dbl))  [unwired: 4 in, 2 out]
        n125 = Multiply(1:w252, 2:w247) -> (0:w235:waveform(dbl)[])  [unwired: 1 in, 1 out]
        n126 = Multiply(1:w246, 2:w247) -> (0:w233:waveform(dbl)[])  [unwired: 1 in, 1 out]
        n127 = Array Size(array=w238) -> (size(s)=w237:i32)
        n128 = Multiply(x=w235, y=2.0 ("amplitude")) -> (x*y=w231:waveform(dbl)[])
        n129 = Multiply(x=w233, y=2.0 ("amplitude")) -> (x*y=w229:waveform(dbl)[])
        n130 = call-poly <vilib>:"Digital IIR Filter.vi"("IIR filter specifications"="IIR filter specifications", "reset filters"="reset filters", "filter structure option"="filter structure option", "signal(s) in"=w231) -> ("signal(s) out"=w245:waveform(dbl)[])  [unwired: 5 in, 2 out]
        n131 = call-poly <vilib>:"Digital IIR Filter.vi"("IIR filter specifications"="IIR filter specifications", "reset filters"="reset filters", "filter structure option"="filter structure option", "signal(s) in"=w229) -> ()  [unwired: 5 in, 3 out]
        n132 = call-poly <vilib>:"Basic Averaged DC-RMS.vi"("reset"="reset filters", "averaging type"="averaging type", "signals in"=w245) -> ("DC values"=w223:dbl[])  [unwired: 5 in, 3 out]
        n133 = case shown="1, Default" w237 {
          tunnel: w238 -> [w280 w286]
          tunnel: [w279 w285] -> w240
          tunnel: w223 -> [w278 _]
          frame 1, Default {
            n134 = for {
              tunnel: w280 -> [w284] mode=indexing
              tunnel: [w282] -> w279 mode=indexing
              tunnel: w278 -> [w281] mode=indexing
              n135 = Build Array(w281, w284) -> (w283:dbl[])
              n136 = Bundle By Name("Y"=w283) -> (w282:waveform(dbl))  [unwired: 1 in]
            }
          }
          frame 0 {
            n137 = for {
              tunnel: w286 -> [w289] mode=indexing
              tunnel: [w287] -> w285 mode=indexing
              n138 = Build Array(w289) -> (w288:dbl[])
              n139 = Bundle By Name("Y"=w288) -> (w287:waveform(dbl))  [unwired: 1 in]
            }
          }
        }
        n140 = call-poly <vilib>:"Basic Averaged DC-RMS.vi"("reset"="reset filters", "averaging type"="long term averaging type", "signals in"=w240) -> ("RMS values"=w236:dbl[])  [unwired: 5 in, 3 out]
        n141 = call-poly <vilib>:"Basic Averaged DC-RMS.vi"("reset"="reset filters", "averaging type"="averaging type", "signals in"=w229) -> ("DC values"=w224:dbl[])  [unwired: 5 in, 3 out]
        n142 = global read "Lock-in Globles Multiple Inputs and Outputs used with FGV.vi" "Stop Lockin"() -> (w274:bool)
        n143 = local read "Measure?"() -> (w258:u16[])
        n144 = Decimate 1D Array(w236) -> ()  [unwired: 2 out]
        n145 = Build Array(w223) -> (→"Waveform Chart":dbl[][])
        n146 = case shown="\"FFT\"" "Tab Control" {
          tunnel: w247 -> [_ w291]
          frame "Input signals", Default {
          }
          frame "FFT" {
            n147 = global read "Lock-in Globles Multiple Inputs and Outputs used with FGV.vi" "Reset Lockin"() -> (w295:bool)
            n148 = call-poly <vilib>:"FFT Power Spectrum and PSD.vi"("averaging parameters"="averaging parameters", "restart averaging (F)"=w295, "dB On (F)"="dB On (F)", "window"="window", "time signals"=w291) -> ("Power Spectrum / PSD"=→"Waveform Graph 2":cluster{"f0":dbl, "df":dbl, "magnitude":dbl[]}[])  [unwired: 3 in, 3 out]
          }
        }
        n149 = global read "Lock-in Globles Multiple Inputs and Outputs used with FGV.vi" "Reset Lockin"() -> (w263:bool)
        n150 = Or(x=w274, y="stop") -> (x .or. y?=w272:bool)
        n151 = Decrement(x="Input Signals") -> (x-1=w265:i16)
        n152 = Select(t=4.0 ("f"), s=w272, f=2.0) -> (s? t:f=w271:dbl)
        n153 = for {
          tunnel: w223 -> [w296] mode=indexing
          tunnel: w224 -> [w298] mode=indexing
          tunnel: [w297] -> w244 mode=indexing
          n154 = Re/Im To Polar(2:w298, 3:w296) -> (0:w301:dbl, 1:w299:dbl)
          n155 = expression code="x * 180/pi"(w301) -> (w300:dbl)
          n156 = Build Array(w296, w298, w299, w300) -> (w297:dbl[])
        }
        "Results (X, Y, R, Theta)" <- w244
        n157 = call "Display.vi"("Results"=w244, "Display"="Display", "Lock-in #"=w265, "Amplifier Settings"=w258) -> ("Display 1"=→"Display 1":string, "Display 2"=→"Display 2":string, "Array"=→"Display X (or R) A":dbl[], "Array 2"=→"Display Y (or Theta) A":dbl[])  [unwired: 3 in]
        n158 = Select(t=5.0, s=w263, f=w271) -> (s? t:f=w269:dbl)
        n159 = call "Results FGV.vi"("Function"=enum16{"write", "read"}."write", "Input Signals"=w244) -> ()  [unwired: 4 in, 2 out]
      }
      frame 4 {
        # "This code stops the AI/AO Tasks, erases them, and ends program execution."
        n160 = local read "AO Task"() -> (w312:refnum<k21>[])
        n161 = local read "AI task"() -> (w314:refnum<k21>[])
        n162 = flat-sequence {
          tunnel: w314 -> [w326]
          tunnel: [w325] -> w313
          tunnel: w312 -> [w325]
          tunnel: [w324] -> w311
          tunnel: w313 -> [w332]
          tunnel: w311 -> [w331]
          tunnel: [w331] -> w310
          tunnel: [w330] -> w309
          frame #0 {
            n163 = for {
              tunnel: w326 -> [w329] mode=indexing
              tunnel: [w327] -> w324 mode=indexing
              n164 = call <vilib>:"DAQmx Stop Task.vi"("task/channels in"=w329) -> ("task out"=w327:refnum<k21>)  [unwired: 13 in, 1 out]
              n165 = Wait (ms)(milliseconds to wait=u32 50) -> ()  [unwired: 1 out]
            }
          }
          frame #1 {
            n166 = for {
              tunnel: w332 -> [w335] mode=indexing
              tunnel: [w333] -> w330 mode=indexing
              n167 = call <vilib>:"DAQmx Stop Task.vi"("task/channels in"=w335) -> ("task out"=w333:refnum<k21>)  [unwired: 13 in, 1 out]
              n168 = Wait (ms)(milliseconds to wait=u32 50) -> ()  [unwired: 1 out]
            }
          }
        }
        n169 = flat-sequence {
          tunnel: w310 -> [w318]
          tunnel: w309 -> [w317]
          tunnel: [w317] -> w308
          tunnel: w308 -> [w321]
          frame #0 {
            n170 = for {
              tunnel: w318 -> [w320] mode=indexing
              n171 = Wait (ms)(milliseconds to wait=u32 50) -> ()  [unwired: 1 out]
              n172 = call <vilib>:"DAQmx Clear Task.vi"("task in"=w320) -> ()  [unwired: 14 in, 1 out]
            }
          }
          frame #1 {
            n173 = for {
              tunnel: w321 -> [w323] mode=indexing
              n174 = call <vilib>:"DAQmx Clear Task.vi"("task in"=w323) -> ()  [unwired: 14 in, 1 out]
              n175 = Wait (ms)(milliseconds to wait=u32 50) -> ()  [unwired: 1 out]
            }
          }
        }
      }
      frame 5 {
        # "This code stops AI/AO tasks, deletes them, and restarts program execution."
        n176 = local read "AO Task"() -> (w342:refnum<k21>[])
        n177 = local read "AI task"() -> (w343:refnum<k21>[])
        n178 = flat-sequence {
          tunnel: w343 -> [w350]
          tunnel: [w349] -> w345
          tunnel: w342 -> [w349]
          tunnel: [w348] -> w344
          tunnel: w345 -> [w356]
          tunnel: w344 -> [w355]
          tunnel: [w355] -> w341
          tunnel: [w354] -> w340
          tunnel: w341 -> [w360]
          tunnel: w340 -> [w361]
          tunnel: [w361] -> w339
          tunnel: w339 -> [w364]
          frame #0 {
            n179 = for {
              tunnel: w350 -> [w353] mode=indexing
              tunnel: [w351] -> w348 mode=indexing
              n180 = Wait (ms)(milliseconds to wait=u32 50) -> ()  [unwired: 1 out]
              n181 = call <vilib>:"DAQmx Stop Task.vi"("task/channels in"=w353) -> ("task out"=w351:refnum<k21>)  [unwired: 13 in, 1 out]
            }
          }
          frame #1 {
            n182 = for {
              tunnel: w356 -> [w359] mode=indexing
              tunnel: [w357] -> w354 mode=indexing
              n183 = Wait (ms)(milliseconds to wait=u32 50) -> ()  [unwired: 1 out]
              n184 = call <vilib>:"DAQmx Stop Task.vi"("task/channels in"=w359) -> ("task out"=w357:refnum<k21>)  [unwired: 13 in, 1 out]
            }
          }
          frame #2 {
            n185 = for {
              tunnel: w360 -> [w363] mode=indexing
              n186 = call <vilib>:"DAQmx Clear Task.vi"("task in"=w363) -> ()  [unwired: 14 in, 1 out]
              n187 = Wait (ms)(milliseconds to wait=u32 50) -> ()  [unwired: 1 out]
            }
          }
          frame #3 {
            n188 = for {
              tunnel: w364 -> [w366] mode=indexing
              n189 = call <vilib>:"DAQmx Clear Task.vi"("task in"=w366) -> ()  [unwired: 14 in, 1 out]
              n190 = Wait (ms)(milliseconds to wait=u32 50) -> ()  [unwired: 1 out]
            }
          }
        }
      }
    }
  }
  n191 = disable-structure shown="Enabled" {
    disable-tunnel: "Stream to disk?" -> [w367 _]
    frame Disabled {
      n192 = case shown="True" w367 {
        frame False {
        }
        frame True {
          w376 = FALSE ("averaging")
          n193 = Index Array() -> ()  [unwired: 9 in, 4 out]
          n194 = call-poly <vilib>:"Decimate (single shot).vi"("averaging"=w376, "decimating factor"="decimating factor") -> ("Decimated Array"=w375:dbl[])  [unwired: 8 in, 1 out]
          n195 = call-poly <vilib>:"Decimate (single shot).vi"("averaging"=w376, "decimating factor"="decimating factor") -> ("Decimated Array"=w374:dbl[])  [unwired: 8 in, 1 out]
          n196 = call-poly <vilib>:"Decimate (single shot).vi"("averaging"=w376, "decimating factor"="decimating factor") -> ("Decimated Array"=w373:dbl[])  [unwired: 8 in, 1 out]
          n197 = call <userlib>:"Read PPMS T and B.vi"() -> ("Field"=w370:dbl, "Temperature"=w371:dbl, "Time"=w372:dbl)  [unwired: 3 in]
          n198 = Build Array(w375, w374, w373) -> (w369:dbl[][])
          n199 = call "Stream_lock_in_data.vi"("Input signal 2"=w369, "decimating factor"="decimating factor", "Field"=w370, "Temperature"=w371, "Time"=w372) -> ()  [unwired: 4 in]
        }
      }
    }
    frame Enabled {
    }
  }
